vi "Generate Enum Decl.vi"(10 "枚举列表":map{u32, string}(c390), 11 "枚举名称":string) -> (3 "枚举声明":string)   [LabVIEW 2020]
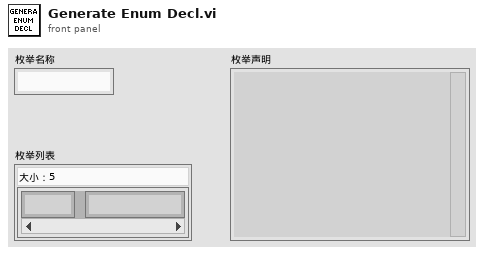
[diagram p1: front panel]
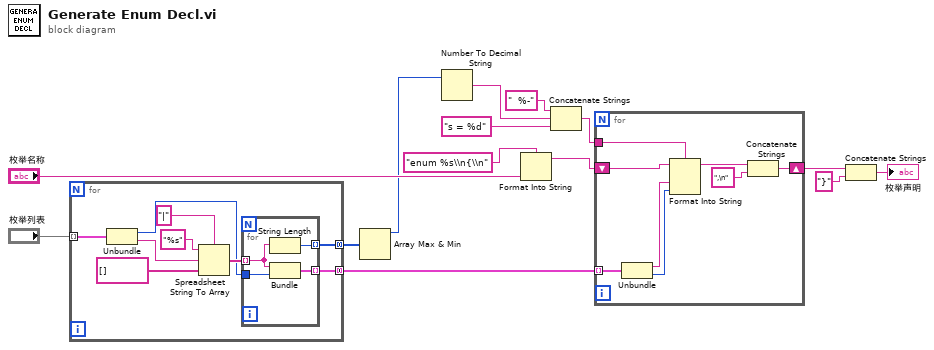
[diagram p0: block diagram]
diagram:
  n1 = for {
    tunnel: "枚举列表" -> [w23] mode=indexing
    tunnel: [w16] -> w6 mode=concatenating
    tunnel: [w15] -> w7 mode=concatenating
    n2 = Unbundle(w23) -> ("key"=w17:u32, "value"=w20:string)
    n3 = Spreadsheet String To Array(delimiter (Tab)="|" ("分隔符(Tab)"), format string="%s" ("格式字符串"), spreadsheet string=w20, array type (2D Dbl)=string[] []) -> (array=w18:string[])
    n4 = for {
      tunnel: w18 -> [w25] mode=indexing
      tunnel: w17 -> [w27]
      tunnel: [w26] -> w16 mode=indexing
      tunnel: [w24] -> w15 mode=indexing
      n5 = String Length(string=w25) -> (length=w24:i32)
      n6 = Bundle(w25, "key"=w27) -> (w26:cluster{string, "key":u32})  [unwired: 1 in]
    }
  }
  n7 = Array Max & Min(array=w7) -> (max value=w4:i32)  [unwired: 3 out]
  n8 = Number To Decimal String(number=w4) -> (decimal integer string=w3:string)  [unwired: 1 in]
  n9 = Format Into String(format string="enum %s\\n{\\n" ("格式字符串"), "枚举名称") -> (resulting string=w1:string)  [unwired: 2 in, 1 out]
  n10 = Concatenate Strings("  %-" ("字符串"), w3, "s = %d" ("格式字符串")) -> (w5:string)
  n11 = for {
    tunnel: w5 -> [w35]
    tunnel: w6 -> [w34] mode=indexing
    shift-right: [w29] -> w2
    shift-left: w1 -> [w31]
    n12 = Unbundle(w34) -> (w33:string, "key"=w32:u32)
    n13 = Format Into String(format string=w35, initial string=w31, w33, w32) -> (resulting string=w28:string)  [unwired: 1 in, 1 out]
    n14 = Concatenate Strings(w28, ",\n" ("字符串")) -> (w29:string)
  }
  n15 = Concatenate Strings(w2, "}" ("字符串")) -> (→"枚举声明":string)
